vi "Set Video Enabled.vi"(8 "error in (no error)":errorcluster, 10 "Video Enabled":bool, 11 "Game Config Panel in":refnum<class "Game Config Panel.lvclass">) -> (0 "error out":errorcluster, 3 "Game Config Panel out":refnum<class "Game Config Panel.lvclass">)   [LabVIEW 2020, in "SB App.lvlib" / "Game Config Panel.lvclass"]
uses:
  Game Config Panel.lvclass
  Game Config Panel.lvclass/Game Config Panel.ctl
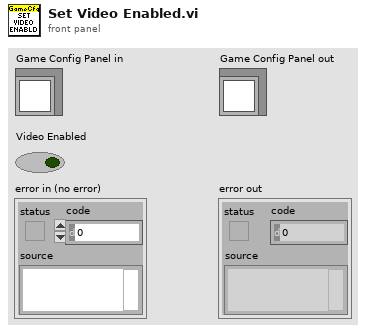
[diagram p1: front panel]
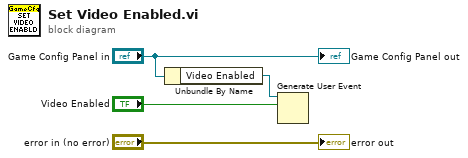
[diagram p0: block diagram]
diagram:
  n1 = Unbundle By Name("Game Config Panel in") -> ("Video Enabled"=w2:refnum<user-event>)
  n2 = Generate User Event(user event=w2, event data cluster="Video Enabled") -> ()  [unwired: 2 in, 2 out]
  "error out" <- "error in (no error)"
  "Game Config Panel out" <- "Game Config Panel in"
